vi "Convert Oval to ROI.vi"(7 "error in (no error)":errorcluster, 10 "Oval Bounds":T2 {"Rotation" min=-90.0 max=90.0 step=1.0 format="%.2f"; "Left" scale=0.0..1024.0; "Right" scale=0.0..1024.0}) -> (0 "error out":errorcluster, 3 "ROI Descriptor":T1 {"Contours"."Type" items=["No Selection", "Point", "Line", "Rectangle", "Oval", "Polygon", "Freehand Region", "Annulus", "Unused2", "Unused3", "Broken Line", "Freehand Line", "Rotated Rectangle"]})   [LabVIEW 2021, in "Image.lvlib"]
doc: "Converts a rectangle or rotated rectangle to an ROI Descriptor. The contour of the ROI Descriptor returned is always of the type rotated rectangle."
uses:
  Image Contour Definition.ctl
  Image Contour ID.ctl
  Image ROI Type.ctl
  Image.lvlib
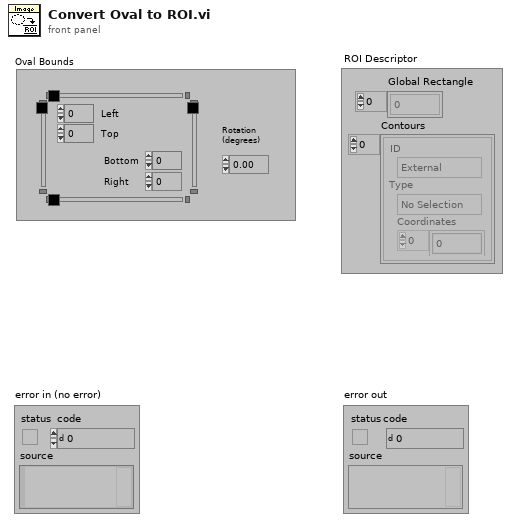
[diagram p1: front panel]
types:
  T1 = typedef "ROI Descriptor" = cluster{"Global Rectangle":i32[], "Contours":cluster{"ID":enum32{"External", "Internal"}, "Type":u32, "Coordinates":i32[]}[]}
  T2 = typedef "IMAQ Rectangle" = cluster{"Left":i32, "Top":i32, "Right":i32, "Bottom":i32, "Rotation":dbl}
  T3 = typedef "Image.lvlib/Image ROI Type.ctl" = enum16{"No Selection", "Point", "Line", "Rectangle", "Oval", "Polygon", "Freehand Region", "Annulus", "Unused2", "Unused3", "Broken Line", "Freehand Line", "Rotated Rectangle"}
  T4 = typedef "Image.lvlib/Image Contour ID.ctl" = enum32{"External", "Internal"}
  T5 = typedef "Image.lvlib/Image Contour Definition.ctl" = cluster{"Contour Type":T4, "ROI Type":T3, "Points":i32[]}
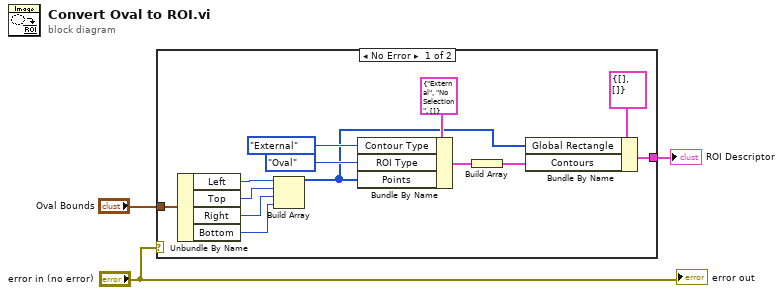
[diagram p0: block diagram]
diagram:
  n1 = case shown="No Error" "error in (no error)" {
    tunnel: [w15 _] -> w3
    tunnel: "Oval Bounds" -> [w11 _]
    frame No Error {
      n2 = Unbundle By Name(w11) -> ("Left"=w10:i32, "Top"=w9:i32, "Right"=w8:i32, "Bottom"=w7:i32)
      n3 = Build Array(w10, w9, w8, w7) -> (w4:i32[])
      n4 = Bundle By Name(cluster=T5 {"Contour Type"=enum."External", "ROI Type"=enum."No Selection", "Points"=[]} ("Contours"), "Contour Type"=Image_Contour_ID."External", "ROI Type"=Image_ROI_Type."Oval", "Points"=w4) -> (w6:T5)
      n5 = Build Array(w6) -> (w5:T5[])
      n6 = Bundle By Name(cluster=T1 {"Global Rectangle"=[], "Contours"=[]} ("Contours"), "Global Rectangle"=w4, "Contours"=w5) -> (w15:T1)
    }
    frame Error {
    }
  }
  "ROI Descriptor" <- w3
  "error out" <- "error in (no error)"
